vi "Store Measuement Config.vi"(8 "error in (no error)":errorcluster, 10 "Measurement Setup Controller.lvlib:Measurement Data.lvclass":refnum<class "Measurement Data.lvclass">, 11 "Measurement Setup in":refnum<class "Measurement Setup.lvclass">) -> (0 "error out":errorcluster, 3 "Measurement Setup out":refnum<class "Measurement Setup.lvclass">)   [LabVIEW 2015, in "Measurement Setup Controller.lvlib" / "Measurement Setup.lvclass"]
uses:
  Measurement Setup.lvclass
  Measurement Data/Measurement Data.lvclass
  Measurement Setup.lvclass/Measurement Setup.ctl
  <vilib>/ActorFramework/Actor/Actor.lvclass/Actor.ctl
  <vilib>/ActorFramework/Message Enqueuer/Message Enqueuer.lvclass/Message Enqueuer.ctl
  <vilib>/ActorFramework/Message Enqueuer/Init from Existing Queue.vi
  <vilib>/ActorFramework/Message Enqueuer/Enqueue.vi
  <vilib>/ActorFramework/Message Priority Queue/Priority Enqueue.vi
  <vilib>/ActorFramework/Stop Msg/Stop Msg.lvclass
  <vilib>/ActorFramework/Message Enqueuer/Message Enqueuer.lvclass
  <vilib>/ActorFramework/Actor/Actor.lvclass
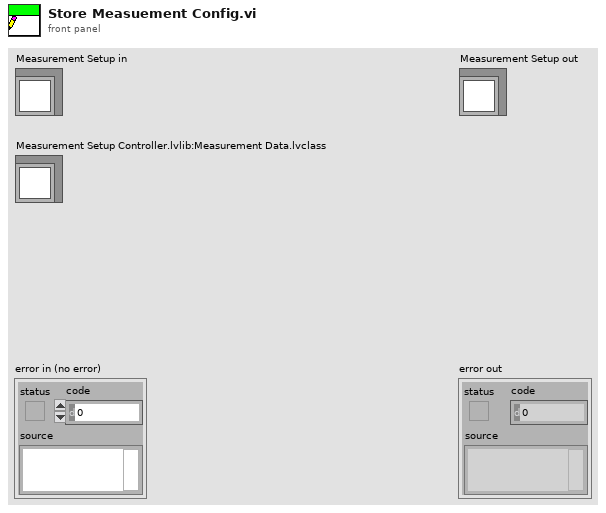
[diagram p1: front panel]
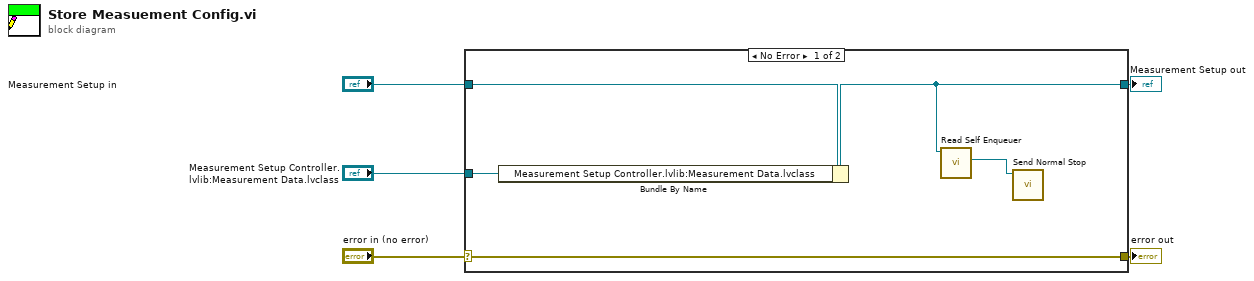
[diagram p0: block diagram]
diagram:
  n1 = case shown="No Error" "error in (no error)" {
    selector: "error in (no error)" -> [w10 w11]
    tunnel: [w10 w11] -> w4
    tunnel: [w7 w12] -> w2
    tunnel: "Measurement Setup in" -> [w9 w12]
    tunnel: "Measurement Setup Controller.lvlib:Measurement Data.lvclass" -> [w8 _]
    frame No Error {
      n2 = Bundle By Name(cluster=w9, "Measurement Setup Controller.lvlib:Measurement Data.lvclass"=w8) -> (w7:refnum<class "Measurement Setup.lvclass">)
      n3 = call <vilib>:"Read Self Enqueuer.vi"("Actor"=w7) -> ("Self Enqueuer"=w6:refnum<class "Message Enqueuer.lvclass">)  [unwired: 10 in]
      n4 = call <vilib>:"Send Normal Stop.vi"("Message Enqueuer"=w6) -> ()  [unwired: 10 in, 1 out]
    }
    frame Error {
    }
  }
  "error out" <- w4
  "Measurement Setup out" <- w2
